vi "M-N随机排列自然数（数组重排）.vi"(1 "M":i32=100, 2 "N":i32=100) -> (0 "M-N-1":i32[](array[numeric]))   [LabVIEW 2012]
doc: "功能：\n\n产生M-N区间自然数随机排列的数组。\n\n\n\ncsxcs_366创建"
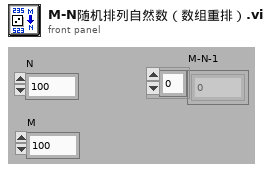
[diagram p1: front panel]
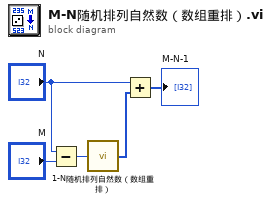
[diagram p0: block diagram]
diagram:
  n1 = Subtract(x="N", y="M") -> (x-y=w3:i32)
  n2 = call "1-N随机排列自然数（数组重排）.vi"("Num (100)"=w3) -> ("1-N"=w4:i32[])
  n3 = Add(x="N", y=w4) -> (x+y=→"M-N-1":i32[])
